vi "Get ENC Pos.vi"(8 "error in (no error)":errorcluster, 11 "FujiMotor in":refnum<class "FujiMotor.lvclass">) -> (0 "error out":errorcluster, 2 "ENC Pos":i32, 3 "FujiMotor out":refnum<class "FujiMotor.lvclass">)   [LabVIEW 2014, in "ALPHA5 RS485.lvlib" / "FujiMotor.lvclass"]
uses:
  FujiMotor.lvclass
  FujiMotor.lvclass/FujiMotor.ctl
  ALPHA5 RS485.lvlib
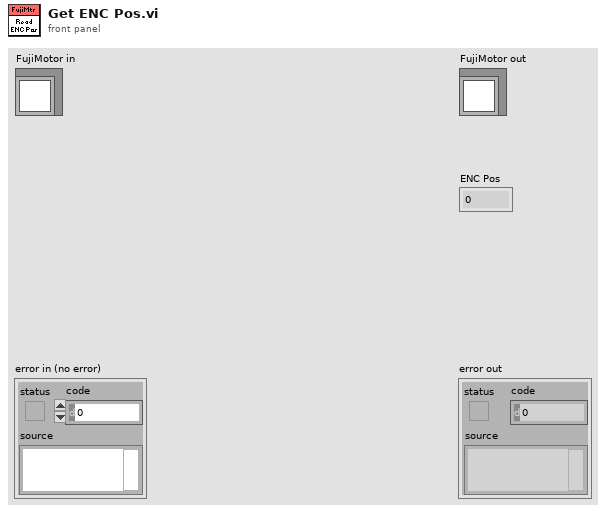
[diagram p1: front panel]
types:
  T1 = typedef "ALPHA5 RS485.lvlib/Port Selection Info.ctl" = cluster{"Port Name":refnum<visa-resource-name>, "Amplifier Num":u8, "Baud Rate":u32, "Char Formation":enum16{"0", "1", "2", "3", "4", "5"}}
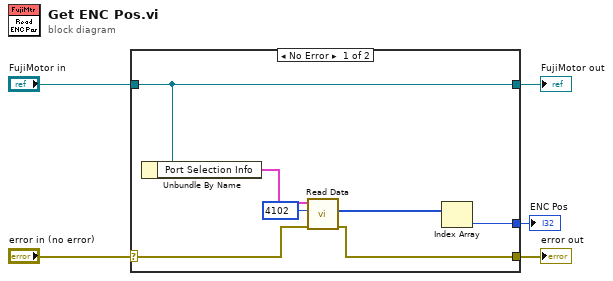
[diagram p0: block diagram]
diagram:
  n1 = case shown="No Error" "error in (no error)" {
    selector: "error in (no error)" -> [w9 w13]
    tunnel: [w8 w13] -> w4
    tunnel: [w12 w14] -> w2
    tunnel: "FujiMotor in" -> [w12 w14]
    tunnel: [w6 _] -> w1
    frame No Error {
      n2 = Unbundle By Name(w12) -> ("Port Selection Info"=w11:T1)
      n3 = call "Read Data.vi"("error in (no error)"=w9, "Address"=u16 4102, "Port Selection Info In"=w11) -> ("error out"=w8:errorcluster, "Data"=w7:u32[])  [unwired: 5 in, 2 out]
      n4 = Index Array(array=w7) -> (element=w6:u32)  [unwired: 1 in]
    }
    frame Error {
    }
  }
  "error out" <- w4
  "FujiMotor out" <- w2
  "ENC Pos" <- w1
